vi "upload_ingest.video.vi"(4 "Properties":map{string, string}(c390), 6 "Labels":string[](array[string]), 7 "Time Stamp":timestamp format="%<%x %.3X>T", 8 "error in":errorcluster, 9 "timeout (ms)":i32=300000, 10 "File Path":path, 11 "Nominal Client in":refnum<class "Nominal Client.lvclass">) -> (0 "error out":errorcluster, 2 "videoRid":string, 3 "Nominal Client out":refnum<class "Nominal Client.lvclass">)   [LabVIEW 2020, in "Nominal Client.lvclass"]
doc: "Uploads a file to S3\nIngests video with common settings:\n - No TimeManifest (uses Start Timestamp and a scale factor of 1.\nNew Target: Name based on path name and timestamp"
uses:
  Nominal Client.lvclass
  datasources/dataset/dataset.lvclass
  nominal types/channelConfig/channelConfig.lvclass
  nominal types/timestampManifest/noManifest/noManifest.lvclass
  C:/sw/labview-client/lv_src/nominal types/timestampManifest/timestampManifest/timestampManifest.lvclass
  datasources/target.video/target.video.lvclass
  C:/sw/labview-client/lv_src/datasources/target/target.lvclass
  datasources/s3/s3.lvclass
  C:/sw/labview-client/lv_src/datasources/source/source.lvclass
  Nominal Client.lvclass/Nominal Client.ctl
  C:/sw/labview-client/lv_src/datasources/payload/payload.lvclass
  C:/sw/labview-client/lv_src/nominal types/timestampManifest/noManifest/noManifest.lvclass
  C:/sw/labview-client/lv_src/datasources/target.video/target.video.lvclass
  C:/sw/labview-client/lv_src/datasources/s3/s3.lvclass
  datasources/target/target.lvclass
  datasources/source/source.lvclass
  nominal types/timestampManifest/timestampManifest.lvlib
  ingest_video.vi
  datasources/source/create_s3.vi
  nominal types/timestampManifest/create.noManifest_scale_factor.vi
  datasources/target.video/create.new_video.vi
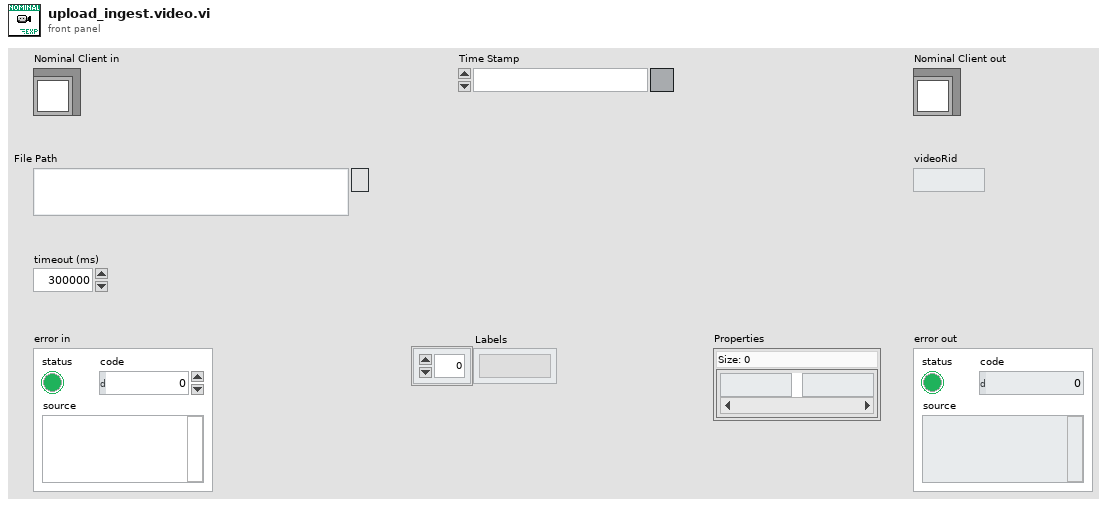
[diagram p1: front panel]
types:
  T1 = cluster{"dataset":refnum<class "dataset.lvclass">, "channelConfig":refnum<class "channelConfig.lvclass">}
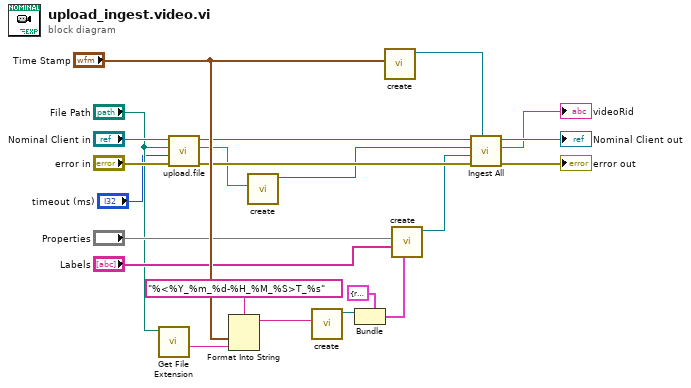
[diagram p0: block diagram]
diagram:
  n1 = call <vilib>:"Get File Extension.vi"("file"="File Path") -> ("filename without extension"=w4:string)  [unwired: 6 in, 4 out]
  n2 = call "upload.file.vi"("error in"="error in", "timeout (ms)"="timeout (ms)", "File"="File Path", "Nominal Client in"="Nominal Client in") -> ("error out"=w20:errorcluster, "Path to S3 File"=w18:string, "Nominal Client out"=w21:refnum<class "Nominal Client.lvclass">)  [unwired: 5 in]
  n3 = Format Into String(format string="%<%Y_%m_%d-%H_%M_%S>T_%s", "Time Stamp", w4) -> (resulting string=w3:string)  [unwired: 2 in, 1 out]
  n4 = call-poly "create.vi"("Path"=w18) -> ("source"=w17:refnum<class "s3.lvclass">)  [unwired: 10 in]
  n5 = call "create.vi"("Name"=w3) -> ("dataset"=w15:refnum<class "dataset.lvclass">)  [unwired: 10 in]
  n6 = Bundle(cluster=T1 {"dataset"=refnum, "channelConfig"=refnum} ("Optional"), "dataset"=w15) -> (w14:T1)  [unwired: 1 in]
  n7 = call-poly "create.vi"("startingTimestamp"="Time Stamp") -> ("Timestamp Manifest"=w2:refnum<class "noManifest.lvclass">)  [unwired: 10 in]
  n8 = call-poly "create.vi"("Optional"=w14, "Labels"="Labels", "Properties"="Properties") -> ("target video"=w19:refnum<class "target.video.lvclass">)  [unwired: 7 in, 1 out]
  n9 = call-poly "Ingest All.vi"("Timestamp Manifest"=w2, "error in"=w20, "Target"=w19, "Source"=w17, "Nominal Client in"=w21) -> ("error out"=→"error out":errorcluster, "videoRid"=→"videoRid":string, "Nominal Client out"=→"Nominal Client out":refnum<class "Nominal Client.lvclass">)  [unwired: 3 in, 1 out]
